vi "Read Instrument.vi"(8 "error in (no error)":errorcluster, 11 "Instrument Sequencer in":refnum<class "Instrument Sequencer.lvclass">) -> (0 "error out":errorcluster, 2 "Instrument Driver":refnum<class "Instrument Driver.lvclass">, 3 "Instrument Sequencer out":refnum<class "Instrument Sequencer.lvclass">)   [LabVIEW 2020, in "Instrument Handler.lvlib" / "Instrument Sequencer.lvclass"]
doc: "Read the Instrument from the Instrument Sequencer."
uses:
  Instrument Sequencer.lvclass
  PPL/HDH.Actor Framework.Core.Instrument Driver.lvlibp/Instrument Driver/Instrument Driver.lvclass
  Instrument Sequencer.lvclass/Instrument Sequencer.ctl
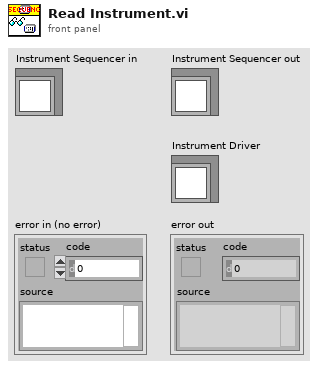
[diagram p1: front panel]
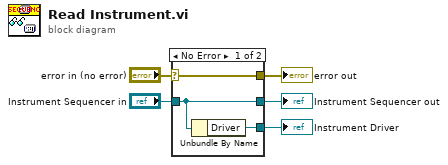
[diagram p0: block diagram]
diagram:
  n1 = case shown="No Error" "error in (no error)" {
    selector: "error in (no error)" -> [w8 w9]
    tunnel: [w8 w9] -> w4
    tunnel: [w6 w10] -> w2
    tunnel: "Instrument Sequencer in" -> [w6 w10]
    tunnel: [w7 _] -> w1
    frame No Error {
      n2 = Unbundle By Name(w6) -> ("Driver"=w7:refnum<class "Instrument Driver.lvclass">)
    }
    frame Error {
    }
  }
  "error out" <- w4
  "Instrument Sequencer out" <- w2
  "Instrument Driver" <- w1
